vi "InsituTestWindow.vi"(8 "error in (no error)":errorcluster, 11 "Instruments in":refnum<class "Instruments.lvclass">) -> (0 "error out":errorcluster, 3 "Instruments out":refnum<class "Instruments.lvclass">)   [LabVIEW 2012, in "Instruments.lvclass"]
uses:
  Instruments.lvclass
  Instruments.lvclass/Instruments.ctl
  SpectrumCommands.ctl
  Controls/SpectrometerOphirSelector.ctl
  SpectrumWindowExit.vi
  <vilib>/Utility/file.llb/Write To Spreadsheet File (DBL).vi
  Controls/Config.ctl
panel:
  in  "first? 2":bool=TRUE
  in  "background":dbl
  out "appended array":dbl[][](array[numeric])
  in  "file path (dialog if empty)":path
  in  "first?":bool=TRUE
  in  "start time":timestamp
  in  "TimeArray":dbl[](array[numeric])
  in  "PowerArray":dbl[](array[numeric])
  in  "WlArray":dbl[](array[numeric])
  in  "VfArray":dbl[](array[numeric])
  in  "Insitu Wl":cluster{"Y":dbl[], "Y":dbl[]}[](graph)
  in  "Insitu Voltage":cluster{"Y":dbl[], "Y":dbl[]}[](graph)
  in  "Insitu Power":cluster{"Y":dbl[], "Y":dbl[]}[](graph)
  in  "Current(mA)":dbl=20.0 min=1.0 max=100.0
  out "Keithley":refnum<visa-resource-name>
  out "DeviceIndicator":bool
  out "Ready":bool
  in  "Int Time(ms)":i32
  in  "Enabled":bool
  in  "Exit":bool
  in  "StopCapture":bool
  in  "StartCapture":bool
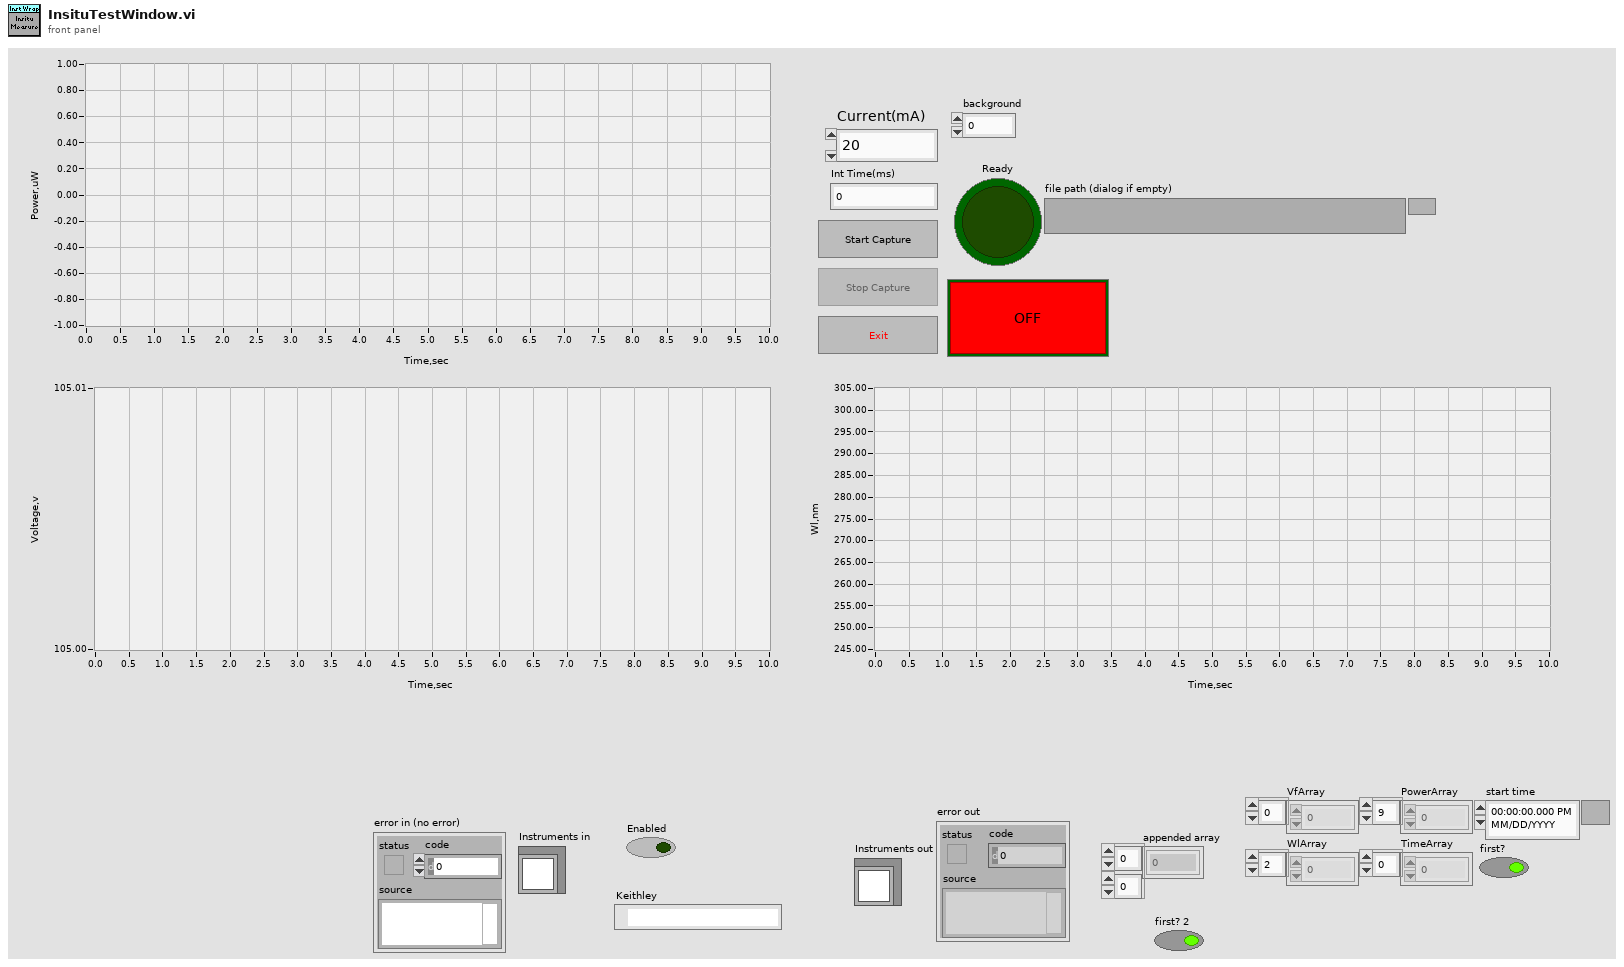
[diagram p1: front panel]
types:
  T1 = enum8{"Enabled", "Disabled", "Disabled and Grayed Out"}
  T2 = cluster{"StopCapture":refnum<vi>, "StartCapture":refnum<vi>, "Exit":refnum<vi>, "Enabled":refnum<vi>, "Ready":refnum<vi>}
  T3 = typedef "Config.ctl" = cluster{"IntTime":i32, "Samples":i32, "PowerMin":dbl, "KneeMin":dbl, "KneeMax":dbl, "Background Wl":dbl, "Settle Delay,ms":u32, "StationId":sgl}
  T4 = typedef "SpectrumCommands.ctl" = enum16{"Init", "StartCapture", "StopCapture", "Calibrate", "TurnDeviceOn", "TurnOffDevice", "Exit"}
  T5 = typedef "SpectrometerOphirSelector.ctl" = enum16{"Get Background", "Measure", "Measure50", "Raw"}
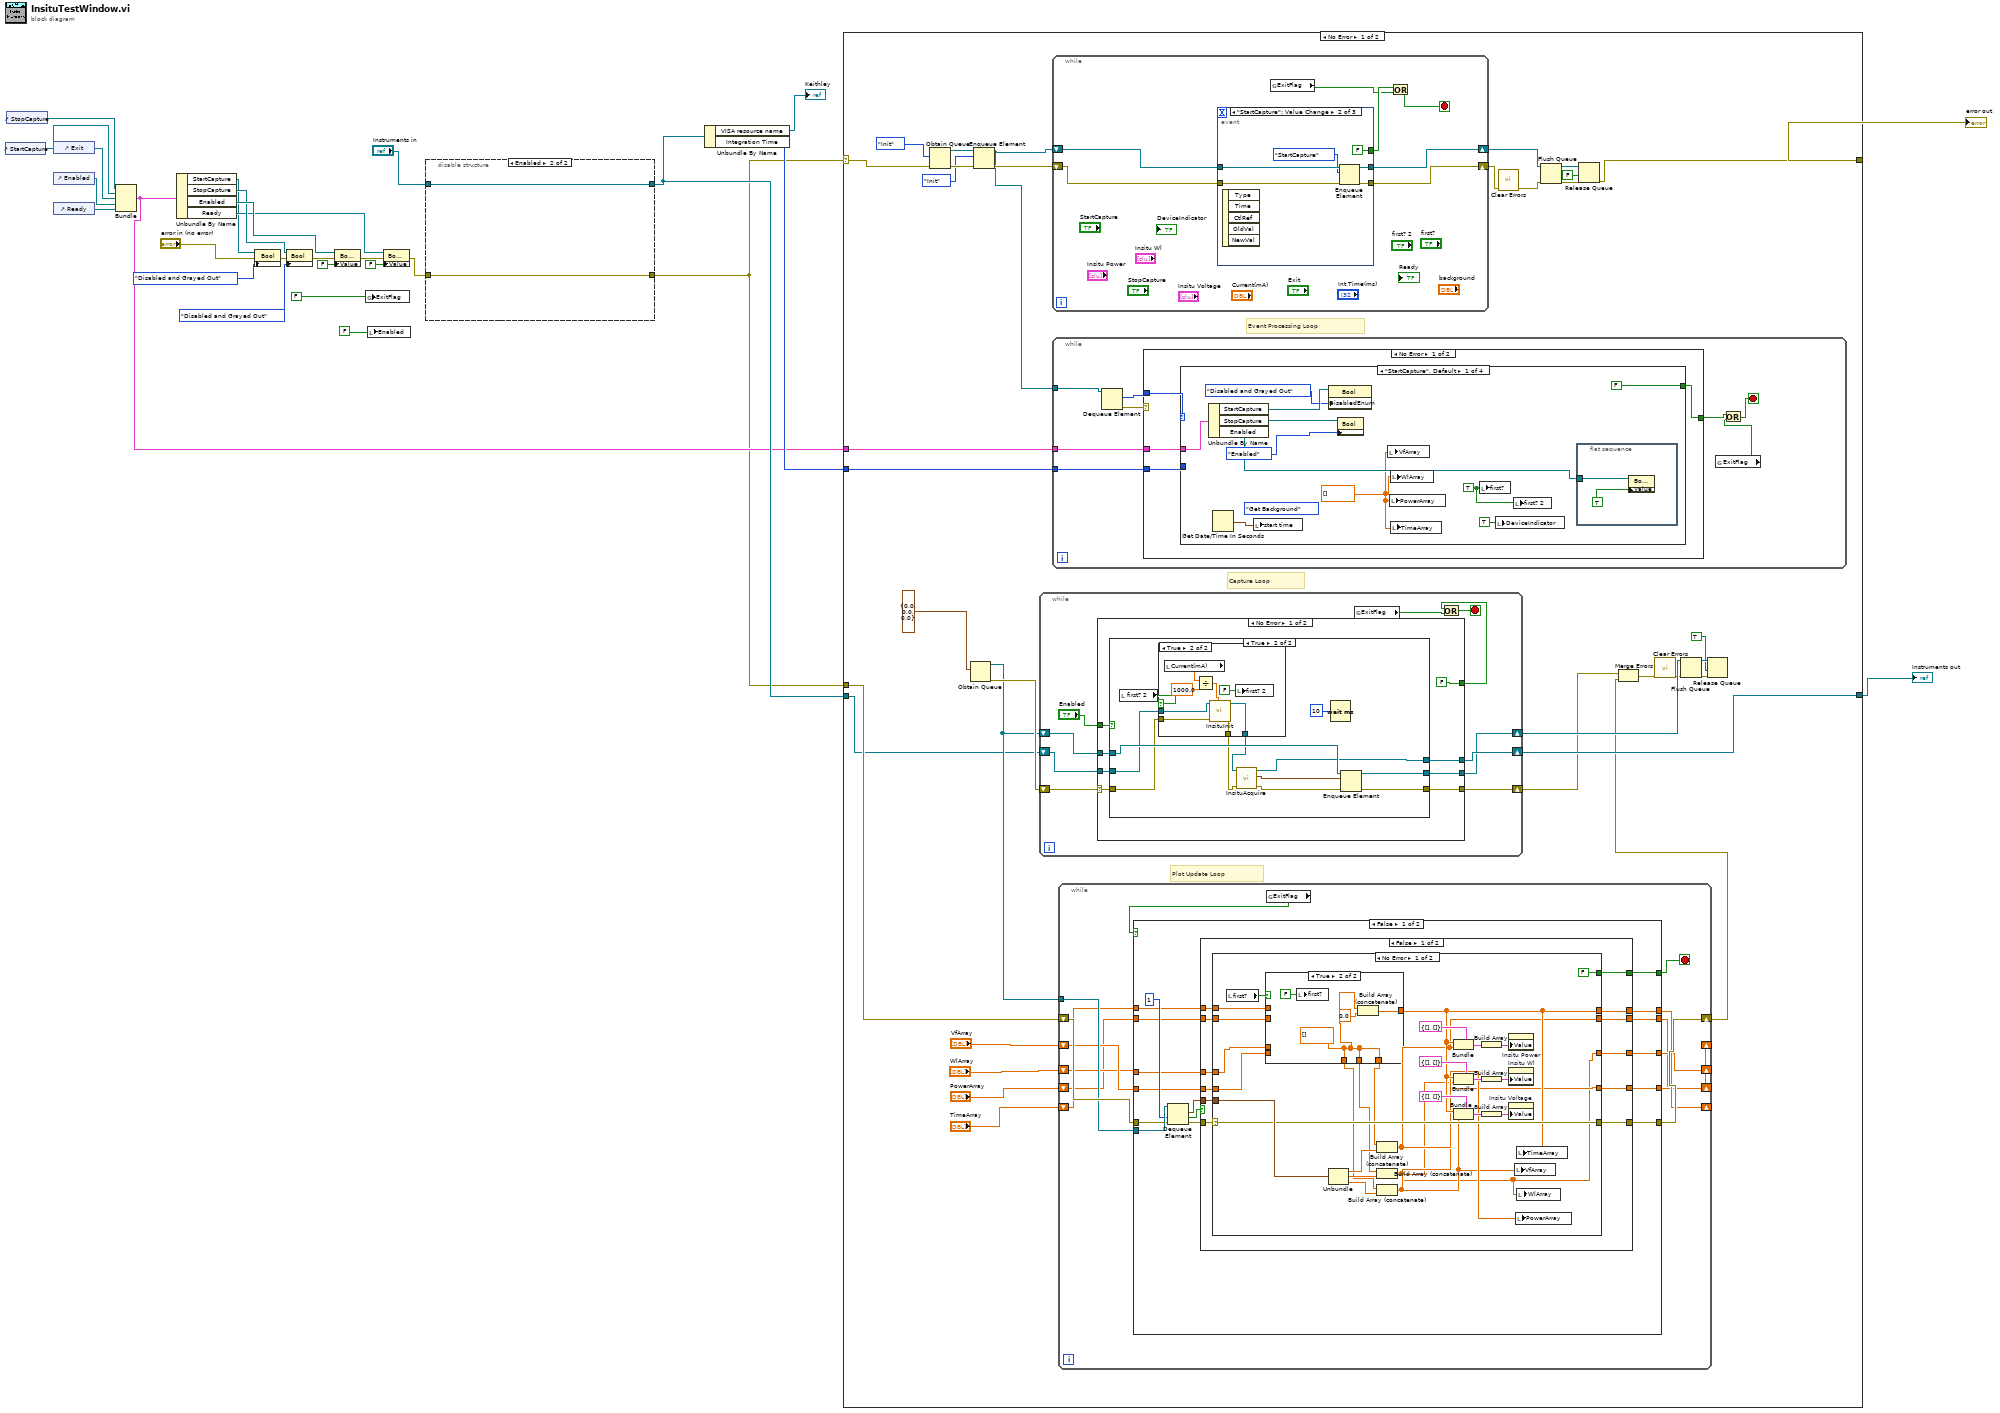
[diagram p0: block diagram]
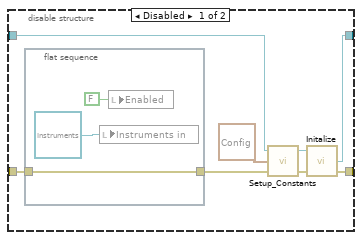
[diagram p2: hidden frame]
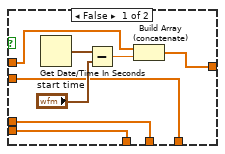
[diagram p3: hidden frame]
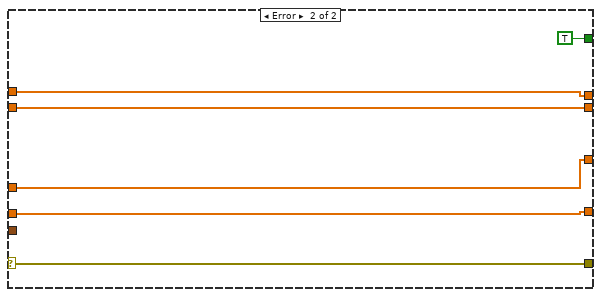
[diagram p4: hidden frame]
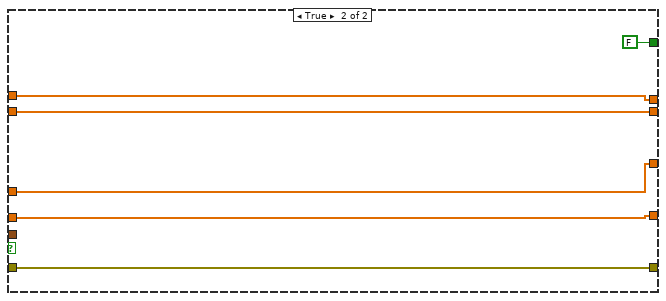
[diagram p5: hidden frame]
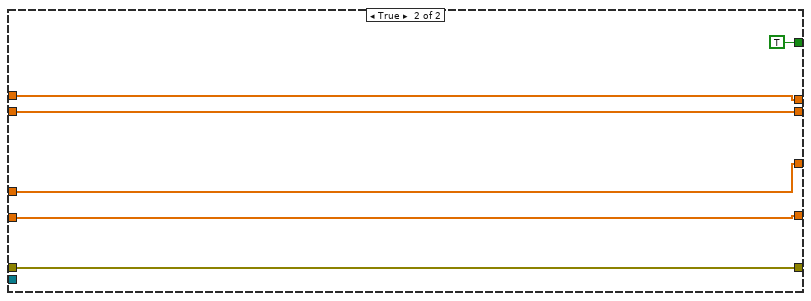
[diagram p6: hidden frame]
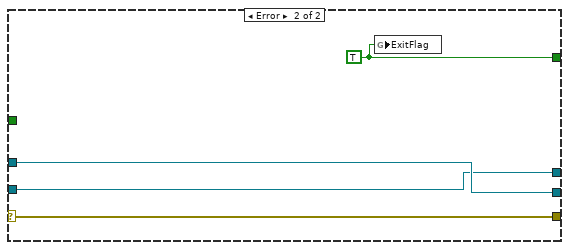
[diagram p9: hidden frame]
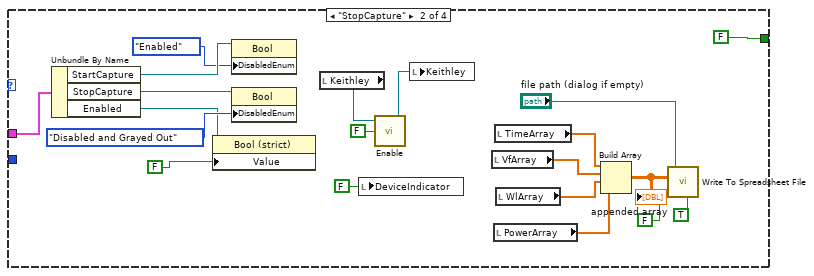
[diagram p10: hidden frame]
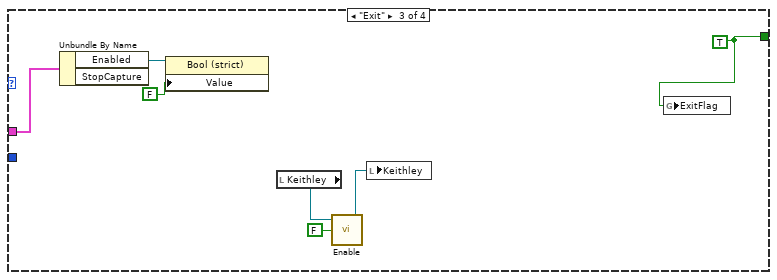
[diagram p11: hidden frame]
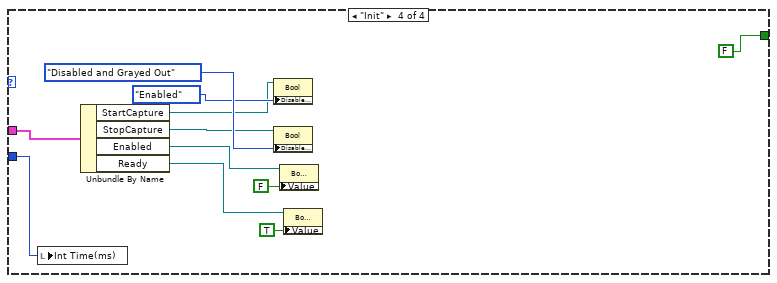
[diagram p12: hidden frame]
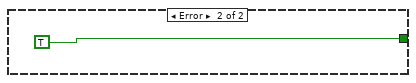
[diagram p13: hidden frame]
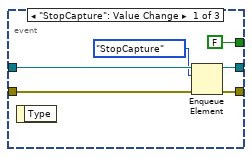
[diagram p14: hidden frame]
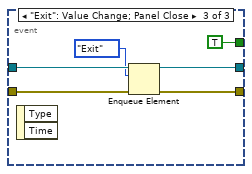
[diagram p15: hidden frame]
diagram:
  n1 = control-ref of="StartCapture"() -> (w25:refnum<vi>)
  n2 = control-ref of="StopCapture"() -> (w26:refnum<vi>)
  n3 = control-ref of="Exit"() -> (w24:refnum<vi>)
  n4 = control-ref of="Enabled"() -> (w23:refnum<vi>)
  n5 = control-ref of="Ready"() -> (w19:refnum<vi>)
  n6 = Bundle("StopCapture"=w26, "StartCapture"=w25, "Exit"=w24, "Enabled"=w23, "Ready"=w19) -> (w6:T2)  [unwired: 1 in]
  n7 = Unbundle By Name(w6) -> ("StartCapture"=w11:refnum<vi>, "StopCapture"=w15:refnum<vi>, "Enabled"=w17:refnum<vi>, "Ready"=w13:refnum<vi>)
  n8 = property class="Bool"(reference=w11, error in="error in (no error)", "DisabledEnum"=T1."Disabled and Grayed Out" ("Disabled")) -> (error out=w9:errorcluster)  [unwired: 1 out]
  n9 = property class="Bool"(reference=w15, error in=w9, "DisabledEnum"=T1."Disabled and Grayed Out" ("Disabled")) -> (error out=w8:errorcluster)  [unwired: 1 out]
  n10 = property class="Bool (strict)"(reference=w17, error in=w8, "Value"=FALSE) -> (error out=w7:errorcluster)  [unwired: 1 out]
  n11 = global write "SpectrumWindowExit.vi" "ExitFlag"(FALSE ("Enabled")) -> ()
  n12 = local write "Enabled"(FALSE ("Enabled")) -> ()
  n13 = property class="Bool (strict)"(reference=w13, error in=w7, "Value"=FALSE) -> (error out=w5:errorcluster)  [unwired: 1 out]
  n14 = disable-structure shown="Enabled" {
    disable-tunnel: [w36 w40] -> w21
    disable-tunnel: [w35 w41] -> w4
    disable-tunnel: "Instruments in" -> [w31 w40]
    disable-tunnel: w5 -> [w29 w41]
    frame Disabled {
      n15 = flat-sequence {
        tunnel: [w38] -> w30
        tunnel: w29 -> [w38]
        frame #0 {
          n16 = local write "Instruments in"(refnum<class "Instruments.lvclass"> refnum ("Instruments in")) -> ()
          n17 = local write "Enabled"(FALSE ("Enabled")) -> ()
        }
      }
      n18 = call-dynamic "Setup_Constants.vi"("error in (no error)"=w30, "Config In"=T3 {"IntTime"=100, "Samples"=3, "PowerMin"=300.0, "KneeMin"=-20.0, "KneeMax"=20.0, "Background Wl"=275.0, "Settle Delay,ms"=0, "StationId"=0.0}, "Instruments in"=w31) -> ("error out"=w32:errorcluster, "Instruments out"=w33:refnum<class "Instruments.lvclass">)  [unwired: 1 in]
      n19 = call-dynamic "Initalize.vi"("error in (no error)"=w32, "Instruments in"=w33) -> ("error out"=w35:errorcluster, "Instruments out"=w36:refnum<class "Instruments.lvclass">)  [unwired: 2 in]
    }
    frame Enabled {
    }
  }
  n20 = Unbundle By Name(w21) -> ("VISA resource name"=→"Keithley":refnum<visa-resource-name>, "Integration Time"=w20:i32)
  n21 = case shown="No Error" w4 {
    selector: w4 -> [w74 w311]
    tunnel: [w66 w311] -> w28
    tunnel: [w72 w310] -> w27
    tunnel: w21 -> [w42 w310]
    tunnel: w6 -> [w48 _]
    tunnel: w4 -> [w70 _]
    tunnel: w20 -> [w50 _]
    frame No Error {
      # "Capture Loop"
      # "Plot Update Loop"
      # "Event Processing Loop"
      n22 = Obtain Queue(element data type=SpectrumCommands."Init", error in (no error)=w74) -> (queue out=w54:refnum<queue>, error out=w53:errorcluster)  [unwired: 3 in, 1 out]
      n23 = Obtain Queue(element data type=cluster{"Power":dbl, "Wl":dbl, "Voltage":dbl} {"Power"=0.0, "Wl"=0.0, "Voltage"=0.0} ("output cluster")) -> (queue out=w71:refnum<queue>, error out=w73:errorcluster)  [unwired: 4 in, 1 out]
      n24 = Enqueue Element(queue=w54, element=SpectrumCommands."Init", error in (no error)=w53) -> (queue out=w49:refnum<queue>, error out=w51:errorcluster)  [unwired: 1 in, 1 out]
      n25 = while {
        shift-right: [w179] -> w61
        shift-left: w71 -> [w180]
        shift-right: [w181] -> w72
        shift-left: w42 -> [w182]
        shift-right: [w178] -> w58
        shift-left: w73 -> [w177]
        stop <- w176 stop-if-true
        n26 = case shown="No Error" w177 {
          selector: w177 -> [w185 w218]
          tunnel: "Enabled" -> [w191 _]
          tunnel: w182 -> [w190 w219]
          tunnel: [w189 w219] -> w181
          tunnel: w180 -> [w188 w220]
          tunnel: [w187 w220] -> w179
          tunnel: [w186 w218] -> w178
          tunnel: [FALSE ("ExitFlag") w217] -> w175
          frame No Error {
            n27 = case shown="True" w191 {
              tunnel: w190 -> [w193 w198]
              tunnel: [w193 w203] -> w189
              tunnel: w188 -> [w194 w206]
              tunnel: [w194 w205] -> w187
              tunnel: [w192 w204] -> w186
              tunnel: w185 -> [w192 w195]
              frame False {
              }
              frame True {
                n28 = local read "first? 2"() -> (w199:bool)
                n29 = case shown="True" w199 {
                  tunnel: w198 -> [w208 w216]
                  tunnel: [w208 w215] -> w197
                  tunnel: [w207 w214] -> w196
                  tunnel: w195 -> [w207 w213]
                  frame False {
                  }
                  frame True {
                    n30 = local read "Current(mA)"() -> (w211:dbl)
                    n31 = Divide(x=w211, y=1000.0) -> (x/y=w209:dbl)
                    n32 = call-dynamic "InsituInit.vi"("Current(A)"=w209, "error in (no error)"=w213, "Instruments in"=w216) -> ("error out"=w214:errorcluster, "Instruments out"=w215:refnum<class "Instruments.lvclass">)  [unwired: 7 in]
                    n33 = local write "first? 2"(FALSE ("first? 2")) -> ()
                  }
                }
                n34 = call-dynamic "InsituAcquire.vi"("error in (no error)"=w196, "Instruments in"=w197) -> ("error out"=w200:errorcluster, "output cluster"=w202:cluster{"Power":dbl, "Wl":dbl, "Voltage":dbl}, "Instruments out"=w203:refnum<class "Instruments.lvclass">)  [unwired: 6 in, 1 out]
                n35 = Wait (ms)(milliseconds to wait=u32 10) -> ()  [unwired: 1 out]
                n36 = Enqueue Element(queue=w206, element=w202, error in (no error)=w200) -> (queue out=w205:refnum<queue>, error out=w204:errorcluster)  [unwired: 1 in, 1 out]
              }
            }
          }
          frame Error {
            w217 = TRUE ("ExitFlag")
            n37 = global write "SpectrumWindowExit.vi" "ExitFlag"(w217) -> ()
          }
        }
        n38 = global read "SpectrumWindowExit.vi" "ExitFlag"() -> (w174:bool)
        n39 = Or(x=w175, y=w174) -> (x .or. y?=w176:bool)
      }
      n40 = while {
        shift-right: [w288] -> w67
        shift-left: w49 -> [w291]
        shift-right: [w289] -> w60
        shift-left: w51 -> [w290]
        stop <- w286 stop-if-true
        n41 = event shown="[1] \"StartCapture\": Value Change" {
          selector: _ -> [_ _ _]
          dyn-events: _ -> [_ _ _]
          timeout: _ -> [_ _ _]
          tunnel: w291 -> [w297 w303 w309]
          tunnel: w290 -> [w296 w302 w308]
          tunnel: [w295 w301 w307] -> w289
          tunnel: [w294 w300 w306] -> w288
          tunnel: [FALSE ("ExitFlag") FALSE ("ExitFlag") TRUE ("ExitFlag")] -> w287
          event "StopCapture": Value Change {
            n42 = event-data() -> ()  [unwired: 1 in, 1 out]
            n43 = Enqueue Element(queue=w297, element=SpectrumCommands."StopCapture", error in (no error)=w296) -> (queue out=w294:refnum<queue>, error out=w295:errorcluster)  [unwired: 1 in, 1 out]
          }
          event "StartCapture": Value Change {
            n44 = event-data() -> ()  [unwired: 1 in, 5 out]
            n45 = Enqueue Element(queue=w303, element=SpectrumCommands."StartCapture", error in (no error)=w302) -> (queue out=w300:refnum<queue>, error out=w301:errorcluster)  [unwired: 1 in, 1 out]
          }
          event "Exit": Value Change; Panel Close {
            n46 = event-data() -> ()  [unwired: 1 in, 2 out]
            n47 = Enqueue Element(queue=w309, element=SpectrumCommands."Exit", error in (no error)=w308) -> (queue out=w306:refnum<queue>, error out=w307:errorcluster)  [unwired: 1 in, 1 out]
          }
        }
        n48 = global read "SpectrumWindowExit.vi" "ExitFlag"() -> (w285:bool)
        n49 = Or(x=w287, y=w285) -> (x .or. y?=w286:bool)
      }
      n50 = while {
        tunnel: w48 -> [w226]
        tunnel: w50 -> [w222]
        tunnel: w49 -> [w221]
        stop <- w224 stop-if-true
        n51 = Dequeue Element(queue=w221) -> (element=w227:T4, error out=w228:errorcluster)  [unwired: 2 in, 2 out]
        n52 = case shown="No Error" w228 {
          tunnel: w227 -> [w232 _]
          tunnel: w226 -> [w231 _]
          tunnel: [w230 TRUE ("x")] -> w225
          tunnel: w222 -> [w229 _]
          frame No Error {
            n53 = case shown="\"StartCapture\", Default" w232 {
              tunnel: w231 -> [w243 w260 w272 w276]
              tunnel: [FALSE ("x") FALSE ("x") w269 FALSE ("x")] -> w230
              tunnel: w229 -> [_ _ _ w282]
              frame "StartCapture", Default {
                (unwired) SpectrometerOphirSelector."Get Background" ("Type")
                w233 = TRUE ("first?")
                w236 = dbl[] [] ("WlArray")
                n54 = Unbundle By Name(w243) -> ("StartCapture"=w242:refnum<vi>, "StopCapture"=w240:refnum<vi>, "Enabled"=w238:refnum<vi>)
                n55 = Get Date/Time In Seconds() -> (seconds since 1Jan1904=w234:timestamp)
                n56 = local write "start time"(w234) -> ()
                n57 = property class="Bool"(reference=w242, "DisabledEnum"=T1."Disabled and Grayed Out" ("Disabled")) -> ()  [unwired: 1 in, 2 out]
                n58 = property class="Bool"(reference=w240, "DisabledEnum"=T1."Enabled" ("Disabled")) -> ()  [unwired: 1 in, 2 out]
                n59 = local write "VfArray"(w236) -> ()
                n60 = local write "PowerArray"(w236) -> ()
                n61 = local write "WlArray"(w236) -> ()
                n62 = local write "TimeArray"(w236) -> ()
                n63 = local write "first?"(w233) -> ()
                n64 = local write "DeviceIndicator"(TRUE ("DeviceIndicator")) -> ()
                n65 = local write "first? 2"(w233) -> ()
                n66 = flat-sequence {
                  tunnel: w238 -> [w245]
                  frame #0 {
                    n67 = property class="Bool (strict)"(reference=w245, "Value"=TRUE) -> ()  [unwired: 1 in, 2 out]
                  }
                }
              }
              frame "StopCapture" {
                n68 = Unbundle By Name(w260) -> ("StartCapture"=w265:refnum<vi>, "StopCapture"=w263:refnum<vi>, "Enabled"=w261:refnum<vi>)
                n69 = property class="Bool (strict)"(reference=w261, "Value"=FALSE) -> ()  [unwired: 1 in, 2 out]
                n70 = property class="Bool"(reference=w265, "DisabledEnum"=T1."Enabled" ("Disabled")) -> ()  [unwired: 1 in, 2 out]
                n71 = property class="Bool"(reference=w263, "DisabledEnum"=T1."Disabled and Grayed Out" ("Disabled")) -> ()  [unwired: 1 in, 2 out]
                n72 = local read "Keithley"() -> (w257:refnum<visa-resource-name>)
                n73 = local write "DeviceIndicator"(FALSE ("DeviceIndicator")) -> ()
                n74 = call "Enable.vi"("Enable Output (T: Enable)"=FALSE, "VISA resource name"=w257) -> ("VISA resource name out"=w256:refnum<visa-resource-name>)  [unwired: 1 in, 1 out]
                n75 = local write "Keithley"(w256) -> ()
                n76 = local read "VfArray"() -> (w252:dbl[])
                n77 = local read "PowerArray"() -> (w250:dbl[])
                n78 = local read "TimeArray"() -> (w253:dbl[])
                n79 = local read "WlArray"() -> (w251:dbl[])
                n80 = Build Array(w253, w252, w251, w250) -> (w249:dbl[][])
                "appended array" <- w249
                n81 = call-poly <vilib>:"Write To Spreadsheet File.vi"("transpose? (no:F)"=TRUE, "append to file? (new file:F)"=FALSE, "2D data"=w249, "file path (dialog if empty)"="file path (dialog if empty)") -> ()  [unwired: 4 in, 1 out]
              }
              frame "Exit" {
                w269 = TRUE ("x")
                n82 = Unbundle By Name(w272) -> ("Enabled"=w271:refnum<vi>)  [unwired: 1 out]
                n83 = property class="Bool (strict)"(reference=w271, "Value"=FALSE) -> ()  [unwired: 1 in, 2 out]
                n84 = local read "Keithley"() -> (w268:refnum<visa-resource-name>)
                n85 = call "Enable.vi"("Enable Output (T: Enable)"=FALSE, "VISA resource name"=w268) -> ("VISA resource name out"=w267:refnum<visa-resource-name>)  [unwired: 1 in, 1 out]
                n86 = local write "Keithley"(w267) -> ()
                n87 = global write "SpectrumWindowExit.vi" "ExitFlag"(w269) -> ()
              }
              frame "Init" {
                n88 = local write "Int Time(ms)"(w282) -> ()
                n89 = Unbundle By Name(w276) -> ("StartCapture"=w273:refnum<vi>, "StopCapture"=w278:refnum<vi>, "Enabled"=w280:refnum<vi>, "Ready"=w275:refnum<vi>)
                n90 = property class="Bool"(reference=w273, "DisabledEnum"=T1."Enabled" ("Disabled")) -> ()  [unwired: 1 in, 2 out]
                n91 = property class="Bool"(reference=w278, "DisabledEnum"=T1."Disabled and Grayed Out" ("Disabled")) -> ()  [unwired: 1 in, 2 out]
                n92 = property class="Bool (strict)"(reference=w280, "Value"=FALSE) -> ()  [unwired: 1 in, 2 out]
                n93 = property class="Bool (strict)"(reference=w275, "Value"=TRUE) -> ()  [unwired: 1 in, 2 out]
              }
            }
          }
          frame Error {
          }
        }
        n94 = global read "SpectrumWindowExit.vi" "ExitFlag"() -> (w223:bool)
        n95 = Or(x=w225, y=w223) -> (x .or. y?=w224:bool)
      }
      n96 = while {
        tunnel: w71 -> [w84]
        shift-right: [w88] -> w57
        shift-left: w70 -> [w86]
        shift-right: [w77] -> _
        shift-left: "VfArray" -> [w83]
        shift-right: [w78] -> _
        shift-left: "WlArray" -> [w82]
        shift-right: [w76] -> _
        shift-left: "PowerArray" -> [w81]
        shift-right: [w79] -> _
        shift-left: "TimeArray" -> [w80]
        stop <- w85 stop-if-true
        n97 = global read "SpectrumWindowExit.vi" "ExitFlag"() -> (w87:bool)
        n98 = case shown="False" w87 {
          tunnel: [w102 w173] -> w88
          tunnel: w86 -> [w99 w173]
          tunnel: [w101 TRUE] -> w85
          tunnel: w84 -> [w100 _]
          tunnel: w83 -> [w96 w171]
          tunnel: w82 -> [w95 w170]
          tunnel: w81 -> [w94 w169]
          tunnel: w80 -> [w93 w168]
          tunnel: [w92 w168] -> w79
          tunnel: [w91 w170] -> w78
          tunnel: [w90 w171] -> w77
          tunnel: [w89 w169] -> w76
          frame False {
            n99 = Dequeue Element(queue=w100, timeout in ms (-1)=1, error in (no error)=w99) -> (element=w103:cluster{"Power":dbl, "Wl":dbl, "Voltage":dbl}, timed out?=w97:bool, error out=w104:errorcluster)  [unwired: 1 out]
            n100 = case shown="False" w97 {
              tunnel: w104 -> [w116 w167]
              tunnel: w103 -> [w115 _]
              tunnel: [w114 w167] -> w102
              tunnel: [w113 FALSE] -> w101
              tunnel: w96 -> [w112 w165]
              tunnel: w95 -> [w111 w164]
              tunnel: w94 -> [w110 w163]
              tunnel: w93 -> [w109 w162]
              tunnel: [w108 w162] -> w92
              tunnel: [w107 w164] -> w91
              tunnel: [w106 w165] -> w90
              tunnel: [w105 w163] -> w89
              frame False {
                n101 = case shown="No Error" w116 {
                  selector: w116 -> [w127 w160]
                  tunnel: w115 -> [w142 _]
                  tunnel: [FALSE TRUE] -> w113
                  tunnel: [w127 w160] -> w114
                  tunnel: w112 -> [w120 w159]
                  tunnel: w111 -> [w119 w158]
                  tunnel: w110 -> [w118 w157]
                  tunnel: w109 -> [w140 w156]
                  tunnel: [w126 w156] -> w108
                  tunnel: [w117 w158] -> w107
                  tunnel: [w124 w159] -> w106
                  tunnel: [w125 w157] -> w105
                  frame No Error {
                    n102 = local read "first?"() -> (w141:bool)
                    n103 = case shown="True" w141 {
                      tunnel: w140 -> [w151 _]
                      tunnel: [w147 w154] -> w126
                      tunnel: [w144 w152] -> w123
                      tunnel: [w145 w152] -> w122
                      tunnel: [w146 w152] -> w121
                      tunnel: w120 -> [w146 _]
                      tunnel: w119 -> [w145 _]
                      tunnel: w118 -> [w144 _]
                      frame False {
                        n104 = Get Date/Time In Seconds() -> (seconds since 1Jan1904=w149:timestamp)
                        n105 = Subtract(x=w149, y="start time") -> (x-y=w150:dbl)
                        n106 = Build Array (concatenate)(w151, w150) -> (w147:dbl[])
                      }
                      frame True {
                        w152 = dbl[] [] ("VfArray")
                        n107 = local write "first?"(FALSE ("first?")) -> ()
                        n108 = Build Array (concatenate)(w152, 0.0) -> (w154:dbl[])
                      }
                    }
                    n109 = Unbundle(w142) -> ("Power"=w128:dbl, "Wl"=w129:dbl, "Voltage"=w130:dbl)
                    n110 = Build Array (concatenate)(w123, w128) -> (w125:dbl[])
                    n111 = Build Array (concatenate)(w122, w129) -> (w117:dbl[])
                    n112 = Build Array (concatenate)(w121, w130) -> (w124:dbl[])
                    n113 = Bundle(cluster=cluster{"Y":dbl[], "Y":dbl[]} {"Y"=[], "Y"=[]}, "Y"=w126, "Y"=w125) -> (w132:cluster{"Y":dbl[], "Y":dbl[]})
                    n114 = Bundle(cluster=cluster{"Y":dbl[], "Y":dbl[]} {"Y"=[], "Y"=[]}, "Y"=w126, "Y"=w117) -> (w138:cluster{"Y":dbl[], "Y":dbl[]})
                    n115 = Bundle(cluster=cluster{"Y":dbl[], "Y":dbl[]} {"Y"=[], "Y"=[]}, "Y"=w126, "Y"=w124) -> (w136:cluster{"Y":dbl[], "Y":dbl[]})
                    n116 = Build Array(w132) -> (w131:cluster{"Y":dbl[], "Y":dbl[]}[])
                    n117 = Build Array(w138) -> (w137:cluster{"Y":dbl[], "Y":dbl[]}[])
                    n118 = Build Array(w136) -> (w134:cluster{"Y":dbl[], "Y":dbl[]}[])
                    n119 = property on="Insitu Power" class="XYGraph (strict)"("Value"=w131) -> ()  [unwired: 2 in, 2 out]
                    n120 = property on="Insitu Wl" class="XYGraph (strict)"("Value"=w137) -> ()  [unwired: 2 in, 2 out]
                    n121 = property on="Insitu Voltage" class="XYGraph (strict)"("Value"=w134) -> ()  [unwired: 2 in, 2 out]
                    n122 = local write "VfArray"(w124) -> ()
                    n123 = local write "PowerArray"(w125) -> ()
                    n124 = local write "TimeArray"(w126) -> ()
                    n125 = local write "WlArray"(w117) -> ()
                  }
                  frame Error {
                  }
                }
              }
              frame True {
              }
            }
          }
          frame True {
          }
        }
      }
      n126 = call <vilib>:"Clear Errors.vi"("error in (no error)"=w60) -> ("error out"=w59:errorcluster)  [unwired: 6 in]
      n127 = Flush Queue(queue=w67, error in (no error)=w59) -> (queue out=w69:refnum<queue>, error out=w68:errorcluster)  [unwired: 1 out]
      n128 = Release Queue(queue=w69, force destroy? (F)=FALSE, error in (no error)=w68) -> (error out=w66:errorcluster)  [unwired: 2 out]
      n129 = Merge Errors(w58, w57) -> (w56:errorcluster)
      n130 = call <vilib>:"Clear Errors.vi"("error in (no error)"=w56) -> ("error out"=w55:errorcluster)  [unwired: 6 in]
      n131 = Flush Queue(queue=w61, error in (no error)=w55) -> (queue out=w64:refnum<queue>, error out=w63:errorcluster)  [unwired: 1 out]
      n132 = Release Queue(queue=w64, force destroy? (F)=TRUE, error in (no error)=w63) -> ()  [unwired: 3 out]
    }
    frame Error {
    }
  }
  "error out" <- w28
  "Instruments out" <- w27
